vi "dfd_Interpret Quantizer.vi"(11 "quantizer":T4={"source"=0, "wl"=16, "iwl"=1, "overflow mode"=enum."Wrap", "rounding mode"=enum."Truncation", "signed?"=TRUE} {"source" items=["Coefficients a/k"=0, "Coefficients b/v"=7, "Input"=1, "Output"=2, "Multiplicand"=3, "Product"=4, "Sum"=5, "Delay"=6]}) -> (1 "rounding mode":T2, 2 "overflow mode":T1, 3 "fxp representation":T3)   [LabVIEW 2017, in "NI_DigFilterLicensed.lvlib"]
uses:
  <vilib>/addons/Digital Filter Design/NI_DigFilterLicensed.lvlib
  <vilib>/addons/Digital Filter Design/_Objects.llb/DFD Quantization Settings.ctl
  <vilib>/addons/Digital Filter Design/_Objects.llb/DFD Quantization Sources.ctl
  <vilib>/fxp/LVFixedPointRepBitsTypeDef.ctl
  <vilib>/fxp/LVFixedPointQuantizationPolicyTypeDef.ctl
  <vilib>/fxp/LVFixedPointOverflowPolicyTypeDef.ctl
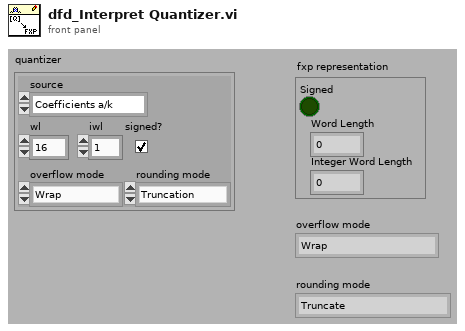
[diagram p1: front panel]
types:
  T1 = typedef "LVFixedPointOverflowPolicyTypeDef.ctl" = enum32{"Wrap", "Saturate"}
  T2 = typedef "LVFixedPointQuantizationPolicyTypeDef.ctl" = enum32{"Truncate", "Round-Half-Up (Asymmetric)", "Round-Half-Even"}
  T3 = typedef "LVFixedPointRepBitsTypeDef.ctl" = cluster{"Signed":bool, "Word Length":u32, "Integer Word Length":i32}
  T4 = typedef "NI_DigFilterLicensed.lvlib/DFD Quantization Settings.ctl" = cluster{"source":T5, "wl":i16, "iwl":i16, "overflow mode":enum16{"Saturation", "Wrap"}, "rounding mode":enum16{"Nearest", "Truncation"}, "signed?":bool}
  T5 = typedef "NI_DigFilterLicensed.lvlib/DFD Quantization Sources.ctl" = u16
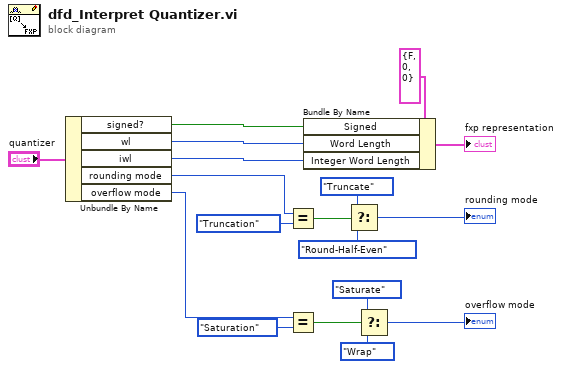
[diagram p0: block diagram]
diagram:
  n1 = Unbundle By Name("quantizer") -> ("signed?"=w16:bool, "wl"=w15:i16, "iwl"=w14:i16, "rounding mode"=w7:enum16{"Nearest", "Truncation"}, "overflow mode"=w6:enum16{"Saturation", "Wrap"})
  n2 = Equal?(x=w7, y=enum16{"Nearest", "Truncation"}."Truncation") -> (x = y?=w11:bool)
  n3 = Equal?(x=w6, y=enum16{"Saturation", "Wrap"}."Saturation") -> (x = y?=w4:bool)
  n4 = Bundle By Name(cluster=T3 {"Signed"=FALSE, "Word Length"=0, "Integer Word Length"=0} ("Fixed-Point Representation:Bits"), "Signed"=w16, "Word Length"=w15, "Integer Word Length"=w14) -> (→"fxp representation":T3)
  n5 = Select(t=LVFixedPointQuantizationPolicyTypeDef."Truncate" ("Quantization"), s=w11, f=LVFixedPointQuantizationPolicyTypeDef."Round-Half-Even" ("Quantization")) -> (s? t:f=→"rounding mode":T2)
  n6 = Select(t=LVFixedPointOverflowPolicyTypeDef."Saturate" ("Fixed-Point:Overflow Policy"), s=w4, f=LVFixedPointOverflowPolicyTypeDef."Wrap" ("Fixed-Point:Overflow Policy")) -> (s? t:f=→"overflow mode":T1)
